vi "Untitled 2 (SubVI).vi"(10 "Analog Input Indexes":u16[](array[numeric]), 11 "Digital in":refnum<vi>) -> (1 "Array":cluster{"start":u16, u16}[](array[cluster]), 2 "start":u16, 3 "Numeric":i32, 4 "stop":i32)   [LabVIEW 2016, in "DNP3_Master_Station_MGCC.lvlib"]
uses:
  DNP3_Master_Station_MGCC.lvlib
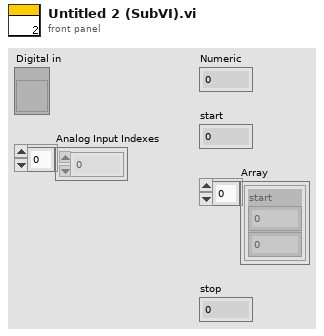
[diagram p1: front panel]
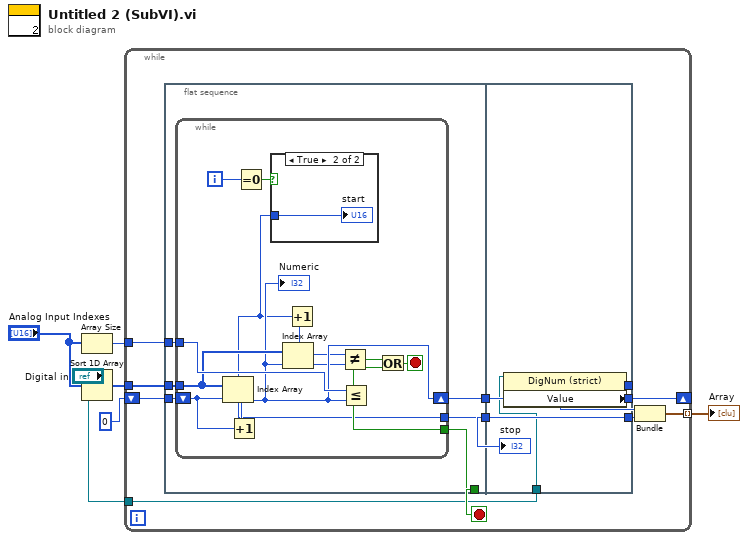
[diagram p0: block diagram]
diagram:
  n1 = Array Size(array="Analog Input Indexes") -> (size(s)=w4:i32)
  n2 = Sort 1D Array(array="Analog Input Indexes") -> (sorted array=w5:u16[])
  n3 = while {
    tunnel: w5 -> [w16]
    tunnel: w4 -> [w17]
    shift-right: [w15] -> _
    shift-left: 0 -> [w14]
    tunnel: [w13] -> w2 mode=indexing
    tunnel: "Digital in" -> [w7]
    stop <- w10 stop-if-true
    n4 = flat-sequence {
      tunnel: w17 -> [w23]
      tunnel: w16 -> [w22]
      tunnel: w14 -> [w20]
      tunnel: [w21] -> w12
      tunnel: [w19] -> w10
      tunnel: [w18] -> w9
      tunnel: [w40] -> w15
      tunnel: w12 -> [w40]
      tunnel: [w39] -> w11
      tunnel: w9 -> [w38]
      tunnel: [w38] -> w8
      tunnel: w7 -> [w37]
      frame #0 {
        n5 = while {
          tunnel: w23 -> [w35]
          tunnel: w22 -> [w28]
          shift-right: [w27] -> w21
          shift-left: w20 -> [w34]
          tunnel: [w29] -> w19
          tunnel: [w24] -> w18
          i -> [w31]
          stop <- w33 stop-if-true
          n6 = Index Array(array=w28, index=w34) -> (element=w24:u16)
          n7 = Increment(x=w34) -> (x+1=w27:i32)
          "Numeric" <- w27
          n8 = Equal To 0?(x=w31) -> (x = 0?=w30:bool)
          n9 = case shown="True" w30 {
            tunnel: w24 -> [_ w36]
            frame False {
            }
            frame True {
              "start" <- w36
            }
          }
          n10 = Index Array(array=w28, index=w27) -> (element=w25:u16)
          n11 = Increment(x=w24) -> (x+1=w26:u16)
          n12 = Not Equal?(x=w26, y=w25) -> (x != y?=w32:bool)
          n13 = Less Or Equal?(x=w35, y=w27) -> (x <= y?=w29:bool)
          n14 = Or(x=w32, y=w29) -> (x .or. y?=w33:bool)
        }
      }
      frame #1 {
        n15 = property class="DigNum (strict)"(reference=w37) -> ("Value"=w39:u16)  [unwired: 1 in, 2 out]
        "stop" <- w38
      }
    }
    n16 = Bundle("Value"=w11, w8) -> (w13:cluster{"Value":u16, u16})  [unwired: 1 in]
  }
  "Array" <- w2
